vi "outputs.vi"() -> ()   [LabVIEW 2018]
panel:
  out "Open":bool
  out "Closed":bool
  out "Open":bool
  out "Closed":bool
  out "Open":bool
  out "Closed":bool
  out "Open":bool
  out "Closed":bool
  out "Open":bool
  out "Closed":bool
  out "Open":bool
  out "data 2":bool[](array[boolean]) caption="data"
  in  "End Loop":bool
  out "error out":errorcluster
  out "task out":refnum<k21>
  in  "device name":tag="Dev1"
  in  "stop (T)":bool=TRUE
  in  "error in":errorcluster
  in  "timeout (s)":dbl=10.0 format="%0.2f"
  in  "data":bool[](array[boolean])
  # "Fuel Gas"
  # "LOx Gas"
  # "Fuel Main"
  # "LOx Main"
  # "Fuel Fill"
  # "LOx Fill"
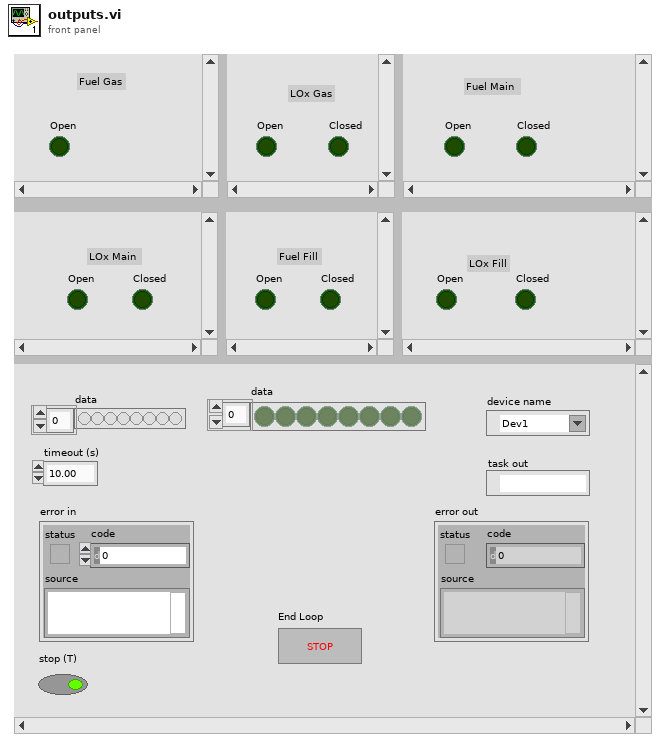
[diagram p1: front panel]
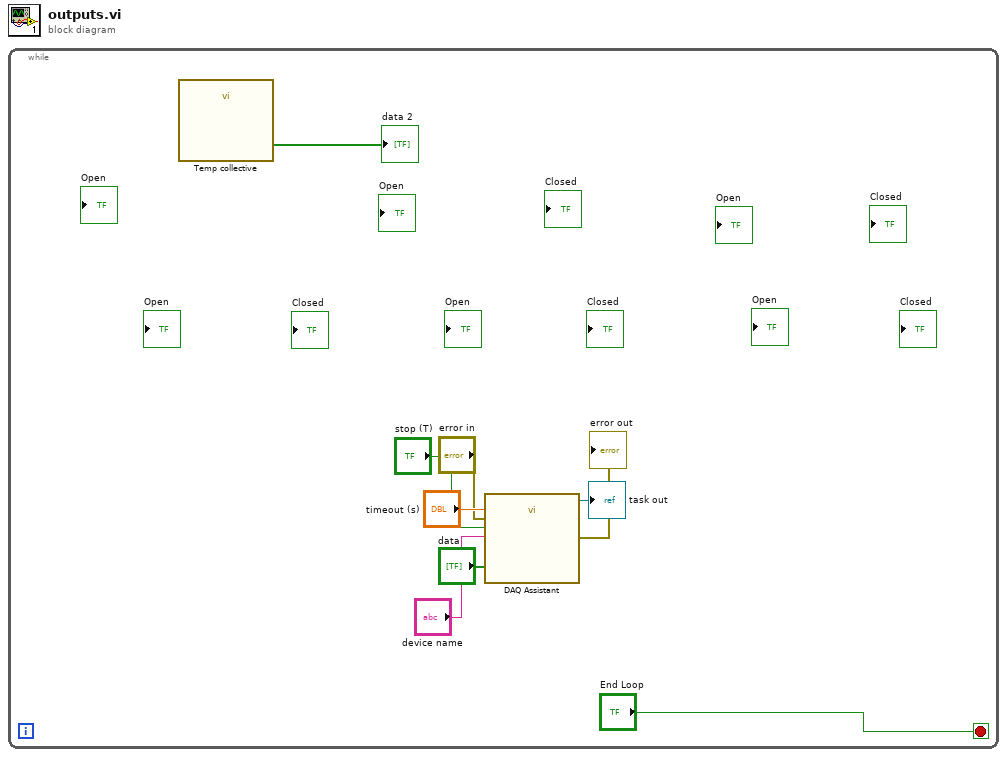
[diagram p0: block diagram]
diagram:
  n1 = while {
    stop <- "End Loop" stop-if-true
    n2 = call "Temp collective"() -> ("data"=→"data 2":bool[])  [unwired: 17 in, 2 out]
    n3 = call "DAQ Assistant"("data"="data", "timeout (s)"="timeout (s)", "error in"="error in", "stop (T)"="stop (T)", "device name"="device name") -> ("task out"=→"task out":refnum<k21>, "error out"=→"error out":errorcluster)  [unwired: 13 in]
  }
